vi "Programa 1.vi"() -> ()   [LabVIEW 2011]
panel:
  out "Multiplicación":dbl
  out "División":dbl
  out "Resta":dbl
  out "Suma":dbl
  in  "Número 2":dbl
  in  "Número 1":dbl
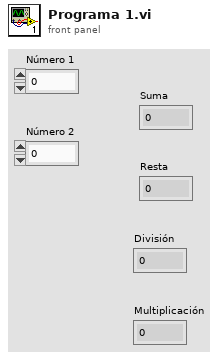
[diagram p1: front panel]
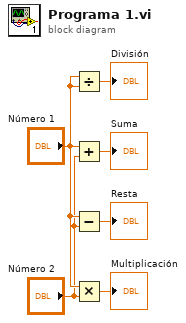
[diagram p0: block diagram]
diagram:
  n1 = Divide(x="Número 1", y="Número 1") -> (x/y=→"División":dbl)
  n2 = Add(x="Número 1", y="Número 2") -> (x+y=→"Suma":dbl)
  n3 = Subtract(x="Número 1", y="Número 2") -> (x-y=→"Resta":dbl)
  n4 = Multiply(x="Número 1", y="Número 2") -> (x*y=→"Multiplicación":dbl)
